vi "Start Cyclic Data Query.vi"(8 "error in (no error)":errorcluster, 10 "Query Period (ms)":i32=1000, 11 "Sensor in":refnum<class "Sensor.lvclass">) -> (0 "error out":errorcluster, 3 "Sensor out":refnum<class "Sensor.lvclass">)   [LabVIEW 2020, in "Sensor.lvlib" / "Sensor.lvclass"]
uses:
  Sensor.lvclass
  C:/Program Files (x86)/National Instruments/LabVIEW 2020/vi.lib/ActorFramework/Actor/Actor.lvclass
  Sensor Messages/Data Query Msg/Data Query Msg.lvclass
  C:/Program Files (x86)/National Instruments/LabVIEW 2020/vi.lib/ActorFramework/Message/Message.lvclass
  Sensor.lvclass/Sensor.ctl
  <vilib>/ActorFramework/Actor/Actor.lvclass/Actor.ctl
  <vilib>/ActorFramework/Message Enqueuer/Message Enqueuer.lvclass/Message Enqueuer.ctl
  <vilib>/ActorFramework/Message Enqueuer/Init from Existing Queue.vi
  <vilib>/ActorFramework/Message Enqueuer/Message Enqueuer.lvclass
  <vilib>/ActorFramework/Actor/Actor.lvclass
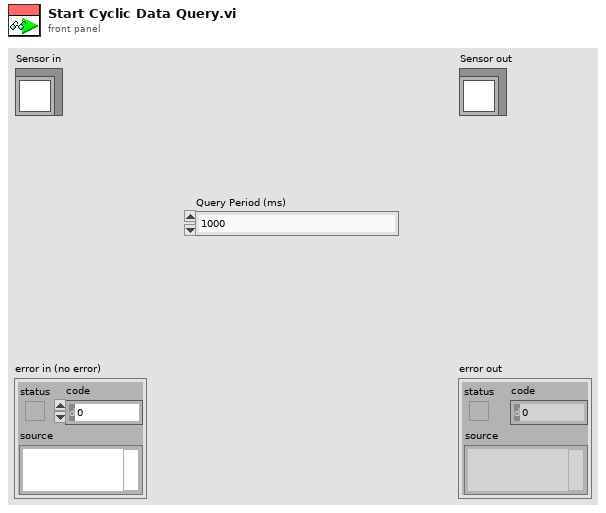
[diagram p1: front panel]
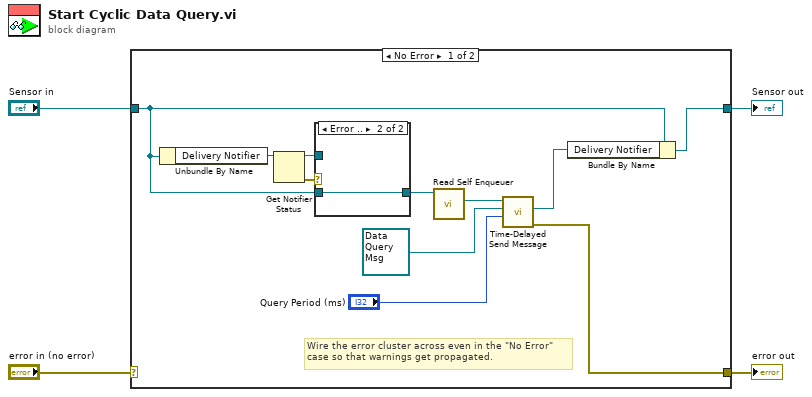
[diagram p0: block diagram]
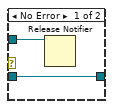
[diagram p2: hidden frame]
diagram:
  n1 = case shown="No Error" "error in (no error)" {
    selector: "error in (no error)" -> [_ w20]
    tunnel: [w9 w20] -> w3
    tunnel: [w15 w19] -> w1
    tunnel: "Sensor in" -> [w6 w19]
    frame No Error {
      # "Wire the error cluster across even in the \"No Error\"\ncase so that warnings get propagated."
      n2 = Unbundle By Name(w6) -> ("Delivery Notifier"=w13:refnum<notifier>)
      n3 = Get Notifier Status(notifier=w13) -> (notifier out=w11:refnum<notifier>, error out=w12:errorcluster)  [unwired: 1 in, 3 out]
      n4 = case shown="Error .." w12 {
        tunnel: w11 -> [w17 _]
        tunnel: [w16 w18] -> w7
        tunnel: w6 -> [w16 w18]
        frame No Error {
          n5 = Release Notifier(notifier=w17) -> ()  [unwired: 2 in, 3 out]
        }
        frame Error {
        }
      }
      n6 = call <vilib>:"Read Self Enqueuer.vi"("Actor"=w7) -> ("Self Enqueuer"=w8:refnum<class "Message Enqueuer.lvclass">)  [unwired: 10 in]
      n7 = call <vilib>:"Time-Delayed Send Message.vi"("Milliseconds To Wait"="Query Period (ms)", "Message"=refnum<class "Data Query Msg.lvclass"> refnum ("Sensor.lvlib:Data Query Msg.lvclass"), "Message Enqueuer"=w8) -> ("error out"=w9:errorcluster, "Delivery Notifier"=w10:refnum<notifier>)  [unwired: 7 in]
      n8 = Bundle By Name(cluster=w6, "Delivery Notifier"=w10) -> (w15:refnum<class "Sensor.lvclass">)
    }
    frame Error {
    }
  }
  "error out" <- w3
  "Sensor out" <- w1
